vi "BlinkingLEDs.vi"(6 "Off Time":dbl, 8 "On Time":dbl, 12 "RED":bool, 13 "GREEN":bool, 14 "BLUE":bool, 15 "Enable?":bool) -> (1 "RED":bool, 2 "GREEN":bool, 3 "BLUE":bool)   [LabVIEW 2016]
uses:
  Common Code/Utilities/TimeManager.vi
  Common Code/Utilities/Toggle.vi
  Common Code/Utilities/Change Detect.vi
  Common Code/Utilities/Change Detect Boolean.vi
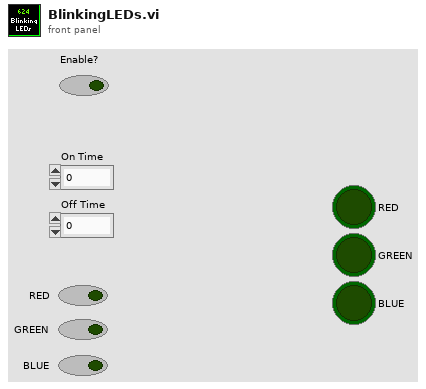
[diagram p1: front panel]
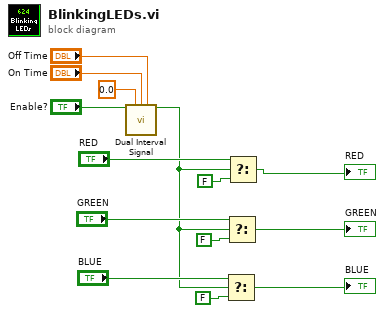
[diagram p0: block diagram]
diagram:
  n1 = call "Dual Interval Signal.vi"("Enable?"="Enable?", "Delay"=0.0, "On Time"="On Time", "Off Time"="Off Time") -> ("Output"=w5:bool)  [unwired: 11 in]
  n2 = Select(t="BLUE", s=w5, f=FALSE) -> (s? t:f=→"BLUE":bool)
  n3 = Select(t="GREEN", s=w5, f=FALSE) -> (s? t:f=→"GREEN":bool)
  n4 = Select(t="RED", s=w5, f=FALSE) -> (s? t:f=→"RED":bool)
